vi "SNED_FLOAT_T_CHANNEL_V_S-1.vi"(1 "数据":dbl) -> (0 "字符串":string)   [LabVIEW 2018]
panel:
  out "4":u8
  out "3":u8
  out "2":u8
  out "1":u8
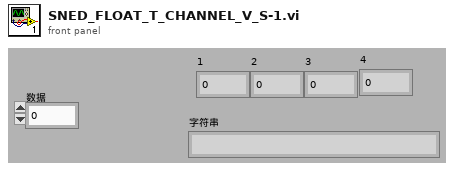
[diagram p1: front panel]
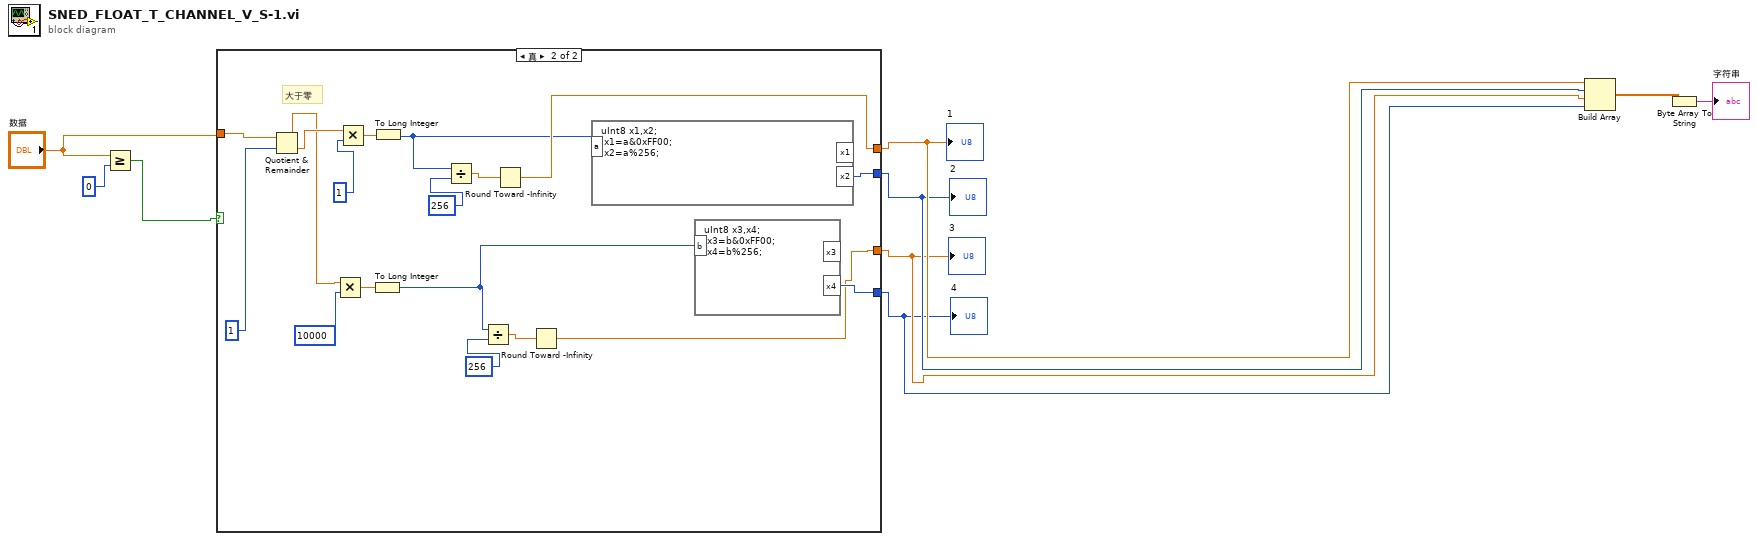
[diagram p0: block diagram]
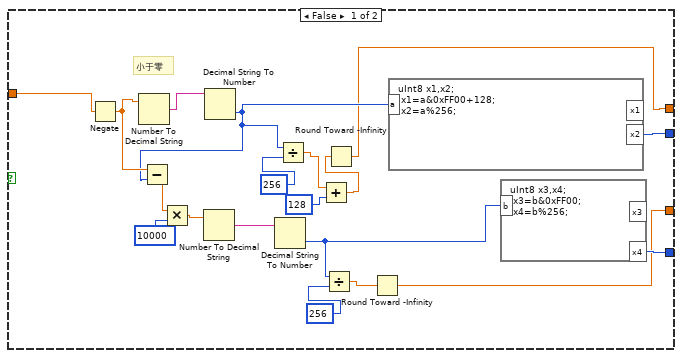
[diagram p2: hidden frame]
diagram:
  n1 = Greater Or Equal?(x="数据", y=0) -> (x >= y?=w2:bool)
  n2 = case shown="真" w2 {
    tunnel: "数据" -> [w24 w38]
    tunnel: [w18 w40] -> w8
    tunnel: [w22 w46] -> w7
    tunnel: [w13 w39] -> w6
    tunnel: [w21 w45] -> w5
    frame False {
      # "小于零"
      n3 = Negate(x=w24) -> (-x=w23:dbl)
      n4 = Number To Decimal String(number=w23) -> (decimal integer string=w25:string)  [unwired: 1 out]
      n5 = Decimal String To Number(string=w25) -> (number=w19:i32)  [unwired: 3 out]
      n6 = Subtract(x=w23, y=w19) -> (x-y=w28:dbl)
      n7 = Multiply(x=w28, y=10000) -> (x*y=w26:dbl)
      n8 = Number To Decimal String(number=w26) -> (decimal integer string=w15:string)  [unwired: 1 out]
      n9 = Decimal String To Number(string=w15) -> (number=w14:i32)  [unwired: 3 out]
      n10 = Divide(x=w19, y=256) -> (x/y=w12:dbl)
      n11 = Add(x=w12, y=128) -> (x+y=w10:dbl)
      n12 = Divide(x=w14, y=256) -> (x/y=w17:dbl)
      n13 = Round Toward -Infinity(1:w10) -> (0:w18:dbl)
      n14 = Round Toward -Infinity(1:w17) -> (0:w13:dbl)
      n15 = formula code="uInt8 x1,x2;\n x1=a&0xFF00+128;\n x2=a%256;"("a"=w19) -> ("x2"=w22:u8)  [unwired: 1 out]
      n16 = formula code="uInt8 x3,x4;\n x3=b&0xFF00;\n x4=b%256;"("b"=w14) -> ("x4"=w21:u8)  [unwired: 1 out]
    }
    frame True {
      # "大于零"
      n17 = Quotient & Remainder(x=w38, y=1) -> (x-y*floor(x/y)=w29:dbl, floor(x/y)=w30:dbl)
      n18 = Multiply(x=w29, y=10000) -> (x*y=w34:dbl)
      n19 = Multiply(x=w30, y=1) -> (x*y=w32:dbl)
      n20 = To Long Integer(number=w34) -> (32bit integer=w31:i32)
      n21 = To Long Integer(number=w32) -> (32bit integer=w33:i32)
      n22 = Divide(x=w33, y=256) -> (x/y=w42:dbl)
      n23 = Divide(x=w31, y=256) -> (x/y=w44:dbl)
      n24 = Round Toward -Infinity(1:w42) -> (0:w40:dbl)
      n25 = Round Toward -Infinity(1:w44) -> (0:w39:dbl)
      n26 = formula code="uInt8 x1,x2;\n x1=a&0xFF00;\n x2=a%256;"("a"=w33) -> ("x2"=w46:u8)  [unwired: 1 out]
      n27 = formula code="uInt8 x3,x4;\n x3=b&0xFF00;\n x4=b%256;"("b"=w31) -> ("x4"=w45:u8)  [unwired: 1 out]
    }
  }
  "1" <- w8
  "2" <- w7
  "3" <- w6
  "4" <- w5
  n28 = Build Array(w8, w7, w6, w5) -> (w9:dbl[])
  n29 = Byte Array To String(unsigned byte array=w9) -> (string=→"字符串":string)
